vi "Vortex SLM.vi"(2 "Action":u16(ring) items=["Read", "Initialize"]) -> (8 "Vortex":dbl[][](array[numeric]))   [LabVIEW 2014]
panel:
  in  "Vortex Rotation":i16=1
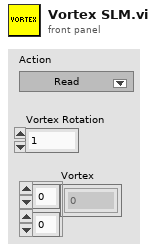
[diagram p1: front panel]
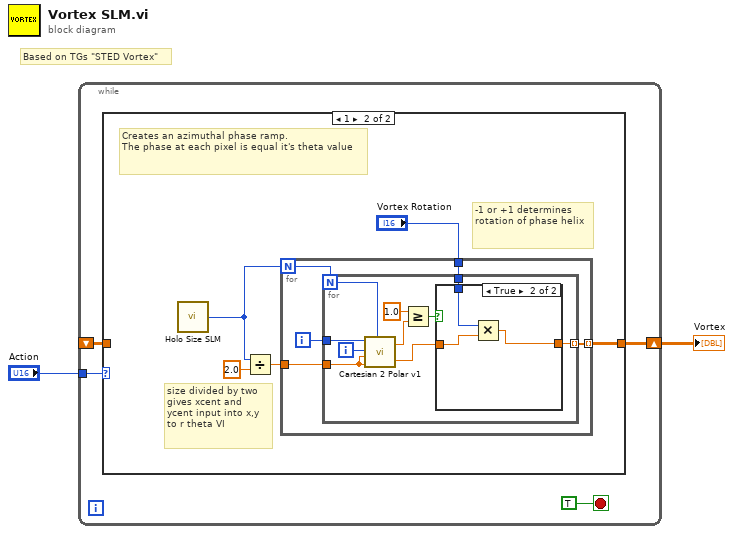
[diagram p0: block diagram]
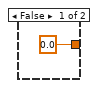
[diagram p3: hidden frame]
diagram:
  # "Based on TGs \"STED Vortex\""
  n1 = while {
    shift-right: [w4] -> w1
    shift-left: _ -> [w3]
    tunnel: "Action" -> [w5]
    stop <- TRUE stop-if-true
    n2 = case shown="1" w5 {
      tunnel: [w7 w9] -> w4
      tunnel: w3 -> [w7 _]
      frame 0, Default {
      }
      frame 1 {
        # "-1 or +1 determines \nrotation of phase helix"
        # "Creates an azimuthal phase ramp.\nThe phase at each pixel is equal it's theta value"
        # "size divided by two gives xcent and ycent input into x,y to r theta VI"
        n3 = call "Holo Size SLM.vi"() -> ("data"=w8:i32)  [unwired: 15 in]
        n4 = Divide(x=w8, y=2.0) -> (x/y=w11:dbl)
        n5 = for {
          N: w8 -> [w14]
          tunnel: [w16] -> w9 mode=indexing
          tunnel: w11 -> [w15]
          tunnel: "Vortex Rotation" -> [w13]
          i -> [w17]
          n6 = for {
            N: w14 -> [w20]
            tunnel: w17 -> [w26]
            tunnel: [w19] -> w16 mode=indexing
            tunnel: w15 -> [w21]
            tunnel: w13 -> [w18]
            i -> [w27]
            n7 = call "Cartesian 2 Polar v1.vi"("x"=w26, "y"=w27, "xcent"=w21, "ycent"=w21, "diam"=w20) -> ("r"=w23:dbl, "t"=w25:dbl)
            n8 = Greater Or Equal?(x=1.0, y=w23) -> (x >= y?=w24:bool)
            n9 = case shown="True" w24 {
              tunnel: w25 -> [_ w31]
              tunnel: [0.0 ("zernike") w29] -> w19
              tunnel: w18 -> [_ w30]
              frame False {
              }
              frame True {
                n10 = Multiply(x=w30, y=w31) -> (x*y=w29:dbl)
              }
            }
          }
        }
      }
    }
  }
  "Vortex" <- w1
